vi "file2str.vi"(1 "Config file path":path) -> (0 "Cmd out":string)   [LabVIEW 2013]
doc: "此VI将config文件中的参数转化为可以直接发送的字符串"
panel:
  out "AfterTreat 2":string[](array[string])
  out "AfterTreat":string[](array[string])
  out "BeforeTreat":string[](array[string])
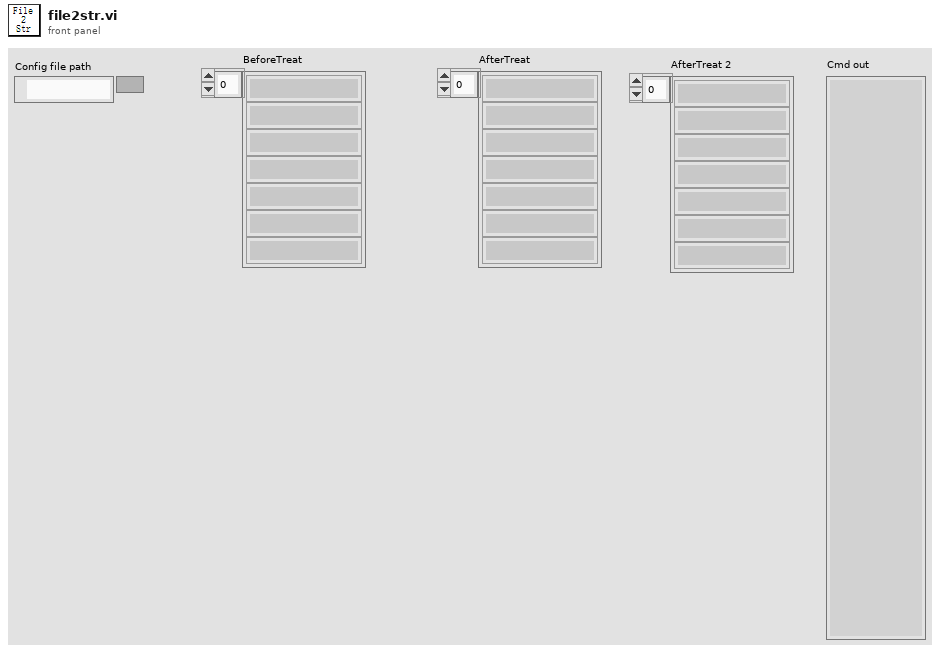
[diagram p1: front panel]
types:
  T1 = enum16{"open", "replace", "create", "open or create", "replace or create", "replace or create with confirmation"}
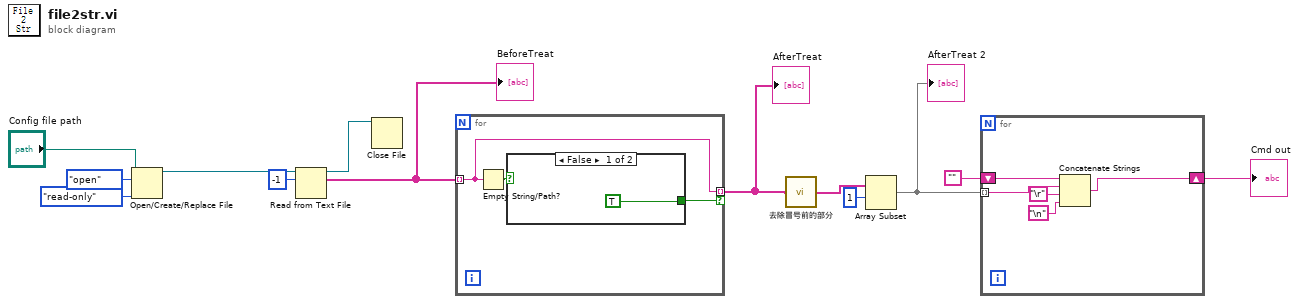
[diagram p0: block diagram]
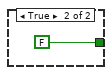
[diagram p2: hidden frame]
diagram:
  n1 = Open/Create/Replace File(file path (use dialog)="Config file path", operation (0:open)=T1."open", access (0:read/write)=enum16{"read/write", "read-only", "write-only"}."read-only") -> (refnum out=w11:refnum<file>)  [unwired: 3 in, 2 out]
  n2 = Read from Text File(file (use dialog)=w11, count=-1) -> (refnum out=w7:refnum<file>, text=w9:string[])  [unwired: 2 in, 2 out]
  "BeforeTreat" <- w9
  n3 = Close File(refnum=w7) -> ()  [unwired: 1 in, 2 out]
  n4 = for {
    tunnel: w9 -> [w15] mode=indexing
    tunnel: [w15] -> w8 mode=indexing if=w14
    n5 = Empty String/Path?(string/path=w15) -> (empty?=w16:bool)
    n6 = case shown="False" w16 {
      tunnel: [TRUE FALSE] -> w14
      frame False {
      }
      frame True {
      }
    }
  }
  "AfterTreat" <- w8
  n7 = call "去除冒号前的部分.vi"("返回值列表"=w8) -> ("返回值参数列表"=w4:string[])
  n8 = Array Subset(array=w4, index=1) -> (w1:string[])  [unwired: 1 in]
  "AfterTreat 2" <- w1
  n9 = for {
    shift-right: [w22] -> w2
    shift-left: "" -> [w23]
    tunnel: w1 -> [w19] mode=indexing
    n10 = Concatenate Strings(w23, w19, "\r", "\n") -> (w22:string)
  }
  "Cmd out" <- w2
